vi "Close Interface.vi"(8 "error in (no error)":errorcluster, 11 "pcap reference":u32) -> (0 "error out":errorcluster)   [LabVIEW 2017, in "lvwpcap.lvlib"]
doc: "This VI closes down the packet sniffing session denoted by pcap reference."
uses:
  lvwpcap.lvlib
  LVpcap.dll
panel:
  # "Select Help»Show Context Help and move the cursor over the VI icon to display help for this VI."
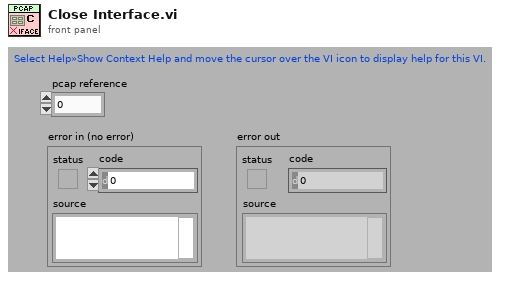
[diagram p1: front panel]
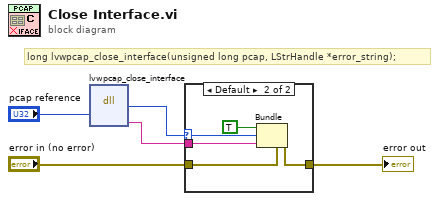
[diagram p0: block diagram]
diagram:
  # "long lvwpcap_close_interface(unsigned long pcap, LStrHandle *error_string);"
  n1 = dll-call lib="C:/Users/Michaello/Desktop/MGR NOWEEEEEEEEEEEEEE/MR PROFINET 2017/Lib/WinPcap/LVpcap.dll" fn="lvwpcap_close_interface"("pcap"="pcap reference") -> ("return type"=w3:i32, "error_string"=w2:string)  [unwired: 5 in, 2 out]
  n2 = case shown="Default" w3 {
    selector: w3 -> [_ w10]
    tunnel: w2 -> [_ w9]
    tunnel: "error in (no error)" -> [w6 w11]
    tunnel: [w6 w7] -> w4
    frame 0 {
    }
    frame Default {
      n3 = Bundle(cluster=w11, "status"=TRUE, "code"=w10, "source"=w9) -> (w7:errorcluster)
    }
  }
  "error out" <- w4
